vi "Area and Perimeter Calculator (Screenshot Recreation).vi"() -> ()   [LabVIEW 2026]
panel:
  out "PERIMETER":dbl
  out "AREA":dbl
  in  "WIDTH":dbl
  in  "HEIGHT":dbl
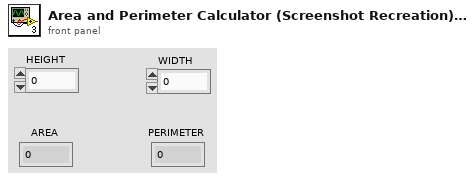
[diagram p1: front panel]
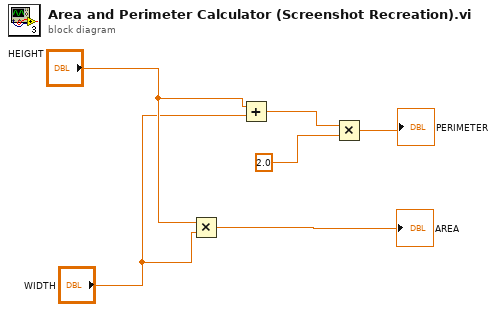
[diagram p0: block diagram]
diagram:
  n1 = Multiply(x="HEIGHT", y="WIDTH") -> (x*y=→"AREA":dbl)
  n2 = Add(x="HEIGHT", y="WIDTH") -> (x+y=w5:dbl)
  n3 = Multiply(x=w5, y=2.0) -> (x*y=→"PERIMETER":dbl)
